vi "Ejector F-B.vi"(1 "Run Forward":bool) -> (0 "Limit Reached":bool)   [LabVIEW 2014]
uses:
  <vilib>/addons/control/pid/pid.llb/PID (DBL).vi
  <vilib>/addons/control/pid/NI_PID_pid.lvlib
panel:
  in  "PID gains":T1={"proportional gain (Kc)"=1.0, "integral time (Ti, min)"=0.01, "derivative time (Td, min)"=0.0} {"derivative time (Td, min)" format="%.3f"; "integral time (Ti, min)" format="%.3f"; "proportional gain (Kc)" format="%.3f"}
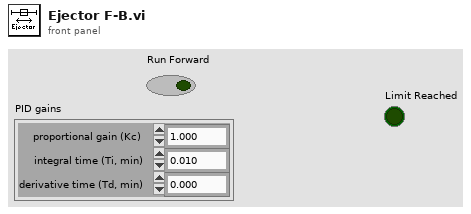
[diagram p1: front panel]
types:
  T1 = cluster{"proportional gain (Kc)":dbl, "integral time (Ti, min)":dbl, "derivative time (Td, min)":dbl}
  T2 = typedef "WPI_EncoderDevRef.ctl" = cluster{"DevStatus":errorcluster, "EncoderIndex":T3, "CounterIndex":T4, "DistancePerCount":dbl, "Decoding Type":T5}
  T3 = typedef "FPGA_EncoderIdx.ctl" = enum8{"Enc 0", "Enc 1", "Enc 2", "Enc 3", "Enc 4", "Enc 5", "Enc 6", "Enc 7", "Invalid"}
  T4 = typedef "FPGA_CounterCtrSystemIndex.ctl" = enum8{"Ctr 0", "Ctr 1", "Ctr 2", "Ctr 3", "Ctr 4", "Ctr 5", "Ctr 6", "Ctr 7", "Invalid"}
  T5 = typedef "WPI_EncoderType.ctl" = enum16{"1x", "2x", "4x"}
  T6 = typedef "WPI_SwitchDevRef.ctl" = cluster{"DevStatus":errorcluster, "DIO Channel":T7, "Controller":T8, "CntIndex":T4, "Normally Closed":bool}
  T7 = typedef "FPGA_DIOChannel.ctl" = enum8{"DIO 0", "DIO 1", "DIO 2", "DIO 3", "DIO 4", "DIO 5", "DIO 6", "DIO 7", "DIO 8", "DIO 9", "DIO MXP 0", "DIO MXP 1", "DIO MXP 2", "DIO MXP 3", "DIO MXP 4", "DIO MXP 5", "DIO MXP 6", "DIO MXP 7", "DIO MXP 8", "DIO MXP 9", "DIO MXP 10", "DIO MXP 11", "DIO MXP 12", "DIO MXP 13", "DIO MXP 14", "DIO MXP 15", "Invalid"}
  T8 = typedef "FPGA_TypedefDigitalModule.ctl" = enum16{"Controller 1"}
  T9 = typedef "WPI_MotorControlDeviceRef.ctl" = cluster{"DeviceStatus":errorcluster, "Type":T10, "PWM":cluster{"Controller":T8, "PWM Channel":T11, "DeadBand":T12}, "CAN":cluster{"Device Number":u8, "Control Mode":T13, "Semaphore":T14, "Max Vout":dbl, "TalonSRX Control Mode":T15}, "Invert":bool, "TransformRef":T16, "InvTransformRef":T16}
  T10 = typedef "WPI_MotorControlType.ctl" = enum16{"PWM", "CAN", "CANTalonSRX"}
  T11 = typedef "FPGA_DIOPWMChannel.ctl" = enum8{"PWM 0", "PWM 1", "PWM 2", "PWM 3", "PWM 4", "PWM 5", "PWM 6", "PWM 7", "PWM 8", "PWM 9", "PWM MXP 0", "PWM MXP 1", "PWM MXP 2", "PWM MXP 3", "PWM MXP 4", "PWM MXP 5", "PWM MXP 6", "PWM MXP 7", "PWM MXP 8", "PWM MXP 9", "Invalid"}
  T12 = typedef "WPI_PWMDeadband.ctl" = cluster{"Name":string, "maxPositivePwm":i32, "minPositivePwm":i32, "centerPwm":i32, "maxNegativePwm":i32, "minNegativePwm":i32, "angularRange":u16}
  T13 = typedef "WPI_CANJaguar_ControlMode.ctl" = enum8{"Percent VBus", "Current", "Speed", "Position", "Voltage"}
  T14 = typedef "Semaphore RefNum" = refnum<k1>
  T15 = typedef "WPI_CANTalonSRX_APIControlMode.ctl" = enum8{"Percent VBus", "Speed", "Position", "Slave", "Unchanged / Invalid"}
  T16 = typedef "WPI_PWMTransform_ConPane.ctl" = refnum<vi>
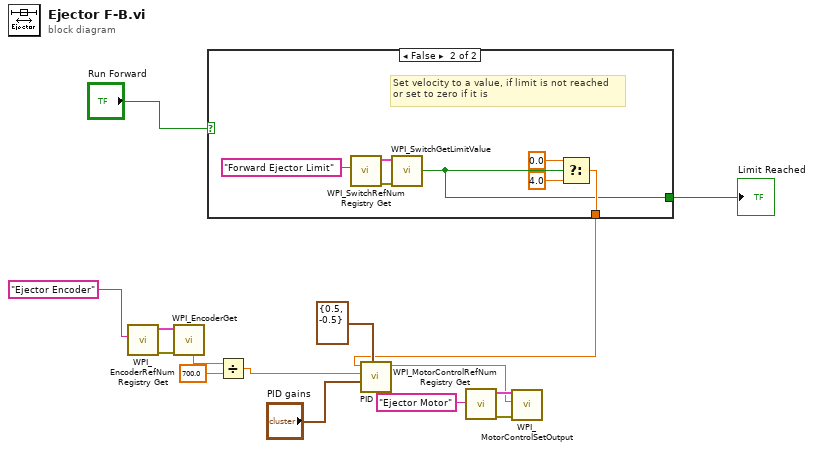
[diagram p0: block diagram]
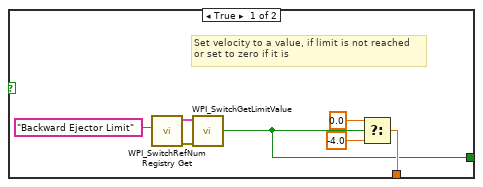
[diagram p2: hidden frame]
diagram:
  n1 = call <vilib>:"WPI_EncoderRefNum Registry Get.vi"("refnum name"="Ejector Encoder") -> ("error out"=w12:errorcluster, "EncoderDevRef"=w11:T2)  [unwired: 9 in]
  n2 = call <vilib>:"WPI_EncoderGet.vi"("error in (no error)"=w12, "EncoderDevRef"=w11) -> ("Rate"=w10:dbl)  [unwired: 4 in, 5 out]
  n3 = case shown="False" "Run Forward" {
    tunnel: [w17 w24] -> w7
    tunnel: [w16 w23] -> w1
    frame True {
      # "Set velocity to a value, if limit is not reached\nor set to zero if it is"
      n4 = call <vilib>:"WPI_SwitchRefNum Registry Get.vi"("refnum name"="Backward Ejector Limit") -> ("error out"=w20:errorcluster, "SwitchDevRef"=w21:T6)  [unwired: 9 in]
      n5 = call <vilib>:"WPI_SwitchGetLimitValue.vi"("error in (no error)"=w20, "SwitchDevRef"=w21) -> ("Switch Pressed"=w16:bool)  [unwired: 7 in, 2 out]
      n6 = Select(t=0.0, s=w16, f=-4.0) -> (s? t:f=w17:dbl)
    }
    frame False {
      # "Set velocity to a value, if limit is not reached\nor set to zero if it is"
      n7 = call <vilib>:"WPI_SwitchRefNum Registry Get.vi"("refnum name"="Forward Ejector Limit") -> ("error out"=w27:errorcluster, "SwitchDevRef"=w28:T6)  [unwired: 9 in]
      n8 = call <vilib>:"WPI_SwitchGetLimitValue.vi"("error in (no error)"=w27, "SwitchDevRef"=w28) -> ("Switch Pressed"=w23:bool)  [unwired: 7 in, 2 out]
      n9 = Select(t=0.0, s=w23, f=4.0) -> (s? t:f=w24:dbl)
    }
  }
  "Limit Reached" <- w1
  n10 = Divide(x=w10, y=700.0) -> (x/y=w8:dbl)
  n11 = call-poly <vilib>:"PID.vi"("output range"=cluster{"output high":dbl, "output low":dbl} {"output high"=0.5, "output low"=-0.5}, "PID gains"="PID gains", "process variable"=w8, "setpoint"=w7) -> ("output"=w3:dbl)  [unwired: 6 in, 1 out]
  n12 = call <vilib>:"WPI_MotorControlRefNum Registry Get.vi"("refnum name"="Ejector Motor") -> ("error out"=w5:errorcluster, "MotorControlDevRef"=w4:T9)  [unwired: 9 in]
  n13 = call <vilib>:"WPI_MotorControlSetOutput.vi"("error in (no error)"=w5, "Output"=w3, "MotorControlDevRef"=w4) -> ()  [unwired: 6 in, 3 out]
